vi "FindPresentationSize.vi"(2 "Pict Refnum":refnum<vi>, 3 "SlideInfo":T1[](array[typedef])) -> (0 "Zoom":dbl, 1 "End":cluster{i16, i16})   [LabVIEW 2014]
uses:
  SlideTypeDef.ctl
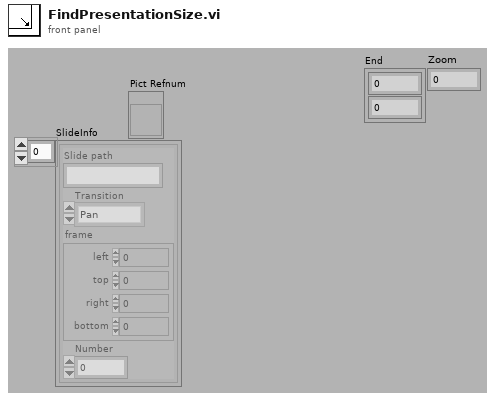
[diagram p1: front panel]
types:
  T1 = typedef "SlideTypeDef.ctl" = cluster{"Slide path":string, "Transition":enum16{"Pan", "Zoom-pan-zoom", "Zoom-wait-Zoom"}, "frame":cluster{"left":i16, "top":i16, "right":i16, "bottom":i16}, "Number":i32}
  T2 = typedef "LVBoundsTypeDef.ctl" = cluster{"Width":u32, "Height":u32}
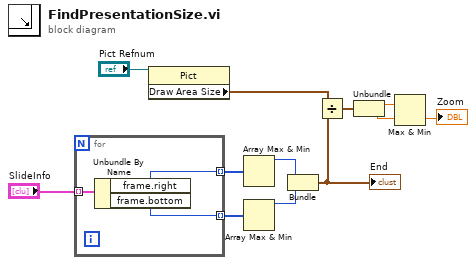
[diagram p0: block diagram]
diagram:
  n1 = for {
    tunnel: "SlideInfo" -> [w15] mode=indexing
    tunnel: [w14] -> w11 mode=indexing
    tunnel: [w13] -> w10 mode=indexing
    n2 = Unbundle By Name(w15) -> ("frame.right"=w14:i16, "frame.bottom"=w13:i16)
  }
  n3 = property class="Pict"(reference="Pict Refnum") -> ("Draw Area Size"=w6:T2)  [unwired: 1 in, 2 out]
  n4 = Array Max & Min(array=w11) -> (max value=w9:i16)  [unwired: 3 out]
  n5 = Array Max & Min(array=w10) -> (max value=w8:i16)  [unwired: 3 out]
  n6 = Bundle(w9, w8) -> (w5:cluster{i16, i16})  [unwired: 1 in]
  "End" <- w5
  n7 = Divide(x=w6, y=w5) -> (x/y=w4:cluster{dbl, dbl})
  n8 = Unbundle(w4) -> (w3:dbl, w2:dbl)
  n9 = Max & Min(x=w3, y=w2) -> (min(x,y)=→"Zoom":dbl)  [unwired: 1 out]
